vi "LowerArm.vi"(8 "error in":errorcluster, 9 "FPGA VI Reference In":T1, 10 "milliseconds to wait \nfor servo to change":u32=100, 11 "Old Angle":dbl) -> (0 "error out":errorcluster, 1 "FPGA VI Reference Out 2":T1, 2 "milliseconds to wait \nfor servo to change Out":u32, 3 "New Angle":dbl)   [LabVIEW 2012]
uses:
  FPGA_ref.ctl
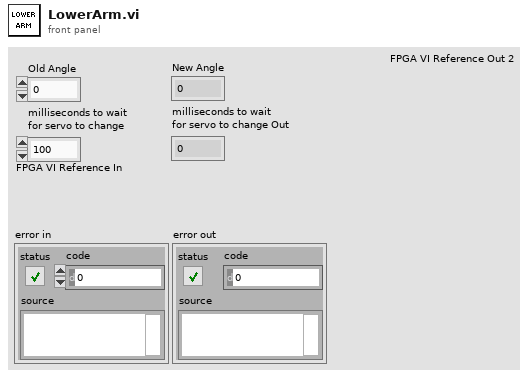
[diagram p1: front panel]
types:
  T1 = typedef "FPGA_ref.ctl" = refnum<k20>
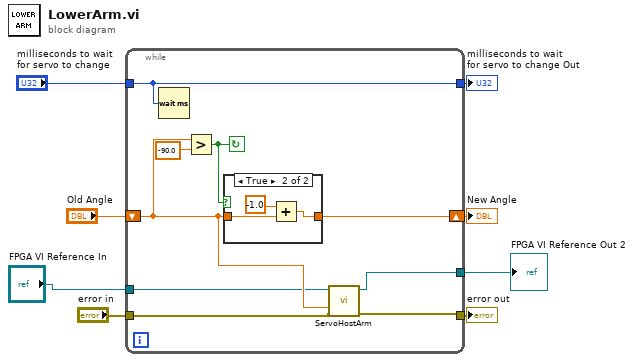
[diagram p0: block diagram]
diagram:
  n1 = while {
    tunnel: "error in" -> [w11]
    shift-right: [w15] -> w5
    shift-left: "Old Angle" -> [w12]
    tunnel: "milliseconds to wait \nfor servo to change" -> [w14]
    tunnel: [w14] -> w4
    tunnel: [w13] -> w3
    tunnel: "FPGA VI Reference In" -> [w10]
    tunnel: [w9] -> w1
    stop <- w16 continue-if-true
    n2 = Wait (ms)(milliseconds to wait=w14) -> ()  [unwired: 1 out]
    n3 = Greater?(x=w12, y=-90.0) -> (0:w16:bool)
    n4 = case shown="True" w16 {
      tunnel: w12 -> [w18 w21]
      tunnel: [w18 w19] -> w15
      frame False {
      }
      frame True {
        n5 = Add(x=-1.0, y=w21) -> (x+y=w19:dbl)
      }
    }
    n6 = call "ServoHostArm.vi"("error in"=w11, "Angle (deg) Arm"=w12, "FPGA VI Reference In"=w10) -> ("error out"=w13:errorcluster, "FPGA VI Reference Out 2"=w9:T1)  [unwired: 7 in]
  }
  "New Angle" <- w5
  "error out" <- w3
  "milliseconds to wait \nfor servo to change Out" <- w4
  "FPGA VI Reference Out 2" <- w1
